vi "Read XY Graph ref.vi"(8 "error in (no error)":errorcluster, 11 "graph_utilities in":refnum<class "graph_utilities.lvclass">) -> (0 "error out":errorcluster, 1 "XY Graph (Control)":refnum<vi>, 2 "XY Graph":refnum<vi>, 3 "graph_utilities out":refnum<class "graph_utilities.lvclass">)   [LabVIEW 2019, in "graph_utilities.lvclass"]
doc: "Read XY Graph control references from the class wire.\n- \"XY Graph\" is the normal target for reading and writing.\n- \"XY Graph (Control)\" is reserved for future use."
uses:
  graph_utilities.lvclass
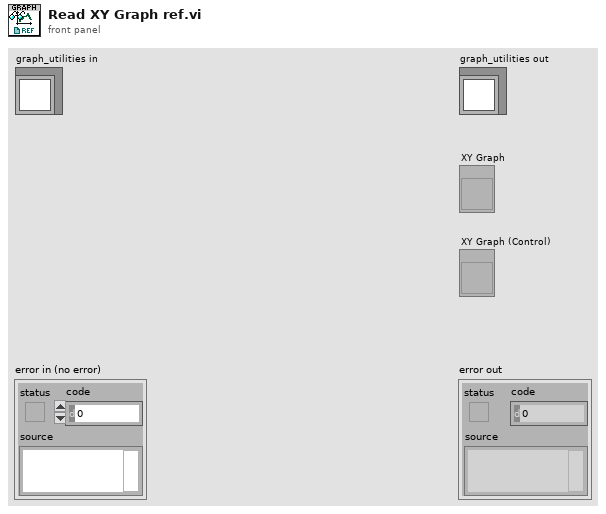
[diagram p1: front panel]
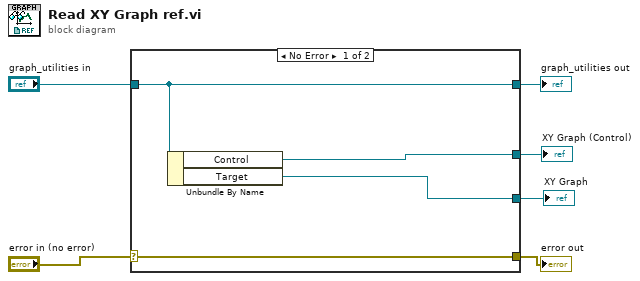
[diagram p0: block diagram]
diagram:
  n1 = case shown="No Error" "error in (no error)" {
    selector: "error in (no error)" -> [w10 w11]
    tunnel: [w10 w11] -> w5
    tunnel: [w9 w12] -> w3
    tunnel: "graph_utilities in" -> [w9 w12]
    tunnel: [w8 _] -> w2
    tunnel: [w7 _] -> w1
    frame No Error {
      n2 = Unbundle By Name(w9) -> ("Control"=w8:refnum<vi>, "Target"=w7:refnum<vi>)
    }
    frame Error {
    }
  }
  "error out" <- w5
  "graph_utilities out" <- w3
  "XY Graph (Control)" <- w2
  "XY Graph" <- w1
